vi "Example.vi"() -> ()   [LabVIEW 2015]
uses:
  <vilib>/Native 3D Graph/xcontrol/3DPC_SurfacePlot.xctl
panel:
  out "3D Graph":refnum<class "Base Datatype.lvclass">[](xcontrol)
  out "new point x":dbl=0.4340593460435067
  out "new point y":dbl=0.8159406539564933
  out "new point z":dbl=0.11811869208701314
  in  "Point 1":cluster{"x":dbl, "y":dbl, "z":dbl, "r":dbl}={"x"=1.0, "y"=0.0, "z"=0.0, "r"=1.0}
  in  "Point 2":cluster{"x":dbl, "y":dbl, "z":dbl, "r":dbl}={"x"=0.0, "y"=1.0, "z"=1.0, "r"=1.0}
  in  "Point 3":cluster{"x":dbl, "y":dbl, "z":dbl, "r":dbl}={"x"=0.0, "y"=0.0, "z"=0.5, "r"=1.0}
  in  "direction":bool
  in  "Stop Button":bool
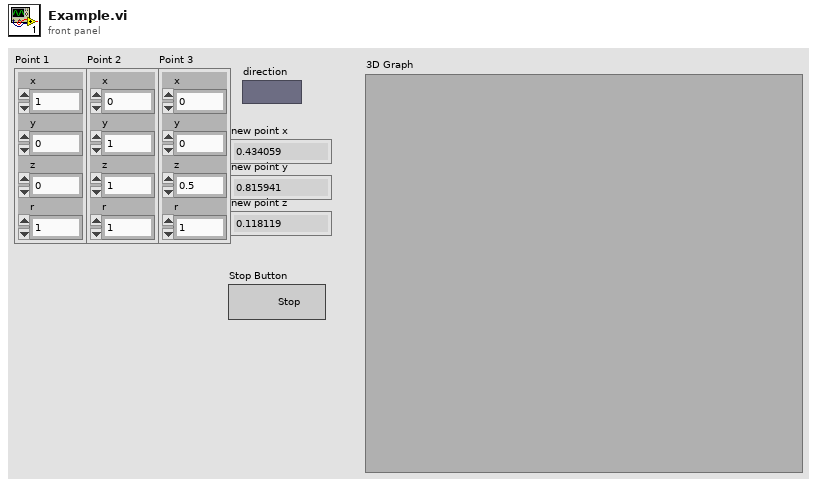
[diagram p1: front panel]
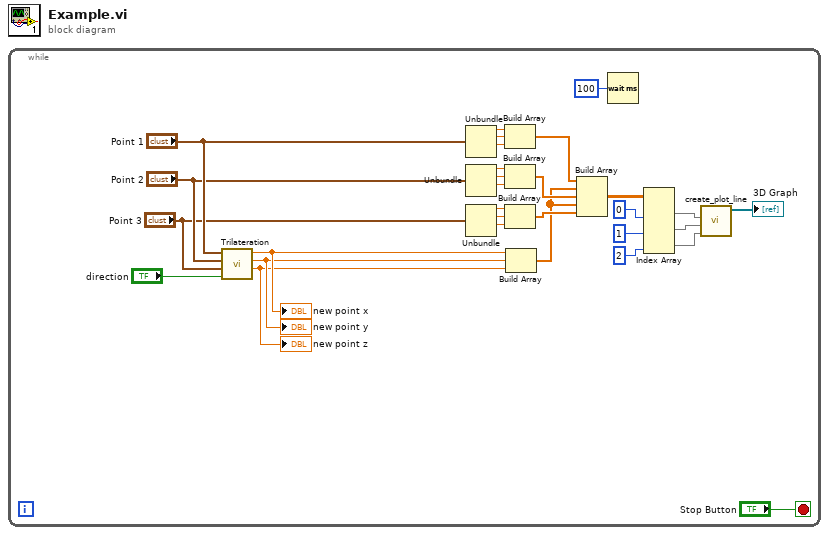
[diagram p0: block diagram]
diagram:
  n1 = while {
    stop <- "Stop Button" stop-if-true
    n2 = call "Trilateration.vi"("direction"="direction", "Point 3"="Point 3", "Point 2"="Point 2", "Point 1"="Point 1") -> ("new point z"=w13:dbl, "new point y"=w14:dbl, "new point x"=w15:dbl)  [unwired: 5 in]
    "new point z" <- w13
    "new point y" <- w14
    "new point x" <- w15
    n3 = Unbundle("Point 1") -> ("x"=w24:dbl, "y"=w22:dbl, "z"=w23:dbl)  [unwired: 1 out]
    n4 = Unbundle("Point 2") -> ("x"=w21:dbl, "y"=w16:dbl, "z"=w17:dbl)  [unwired: 1 out]
    n5 = Unbundle("Point 3") -> ("x"=w20:dbl, "y"=w19:dbl, "z"=w18:dbl)  [unwired: 1 out]
    n6 = Build Array(w24, w22, w23) -> (w12:dbl[])
    n7 = Build Array(w21, w16, w17) -> (w4:dbl[])
    n8 = Build Array(w20, w19, w18) -> (w3:dbl[])
    n9 = Build Array(w15, w14, w13) -> (w2:dbl[])
    n10 = Build Array(w12, w2, w4, w2, w3) -> (w1:dbl[][])
    n11 = Wait (ms)(milliseconds to wait=u32 100) -> ()  [unwired: 1 out]
    n12 = Index Array(array=w1, index (col) #1=0 ("disabled index (col)"), index (col) #2=1 ("disabled index (col)"), index (col) #3=2 ("disabled index (col)")) -> (element #1=w7:dbl[], element #2=w6:dbl[], element #3=w5:dbl[])  [unwired: 3 in]
    n13 = call <vilib>:"create_plot_line.vi"("z vector"=w5, "y vector"=w6, "x vector"=w7) -> ("plots out"=→"3D Graph":refnum<class "Base Datatype.lvclass">[])  [unwired: 2 in, 6 out]
  }
